vi "SQ Hi--C1.vi"(8 "Command Info In":T2, 10 "Sq. Hi--C1":T1, 11 "Scale":string) -> (0 "Command Info Out":T2)   [LabVIEW 2017]
uses:
  <vilib>/Rock Robotics/WPI/Framework/Command Status Info.ctl
  <vilib>/Rock Robotics/WPI/Framework/Completion Status.ctl
  <vilib>/Rock Robotics/WPI/Framework/Completion Notifier.ctl
  Block Clusters/SQ Hi--C1.ctl
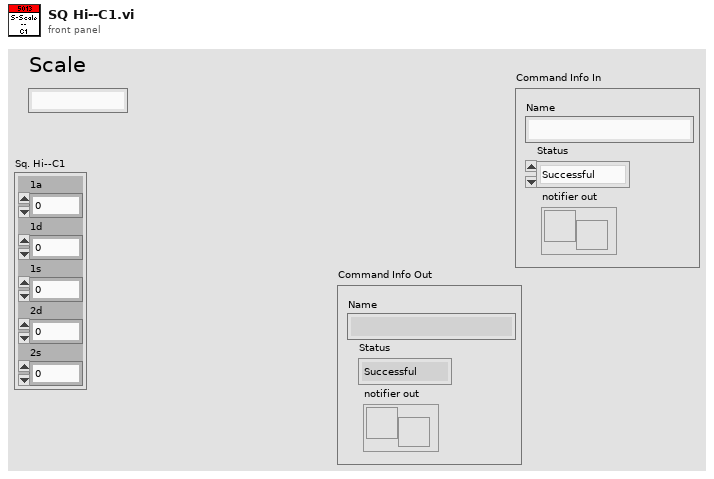
[diagram p1: front panel]
types:
  T1 = typedef "SQ Hi--C1.ctl" = cluster{"1a":dbl, "1d":dbl, "1s":dbl, "2d":dbl, "2s":dbl}
  T2 = typedef "Command Status Info.ctl" = cluster{"Name":string, "Status":T3, "notifier out":T4}
  T3 = typedef "Completion Status.ctl" = enum16{"Successful", "Aborted", "Incomplete"}
  T4 = typedef "Completion Notifier.ctl" = refnum<notifier>
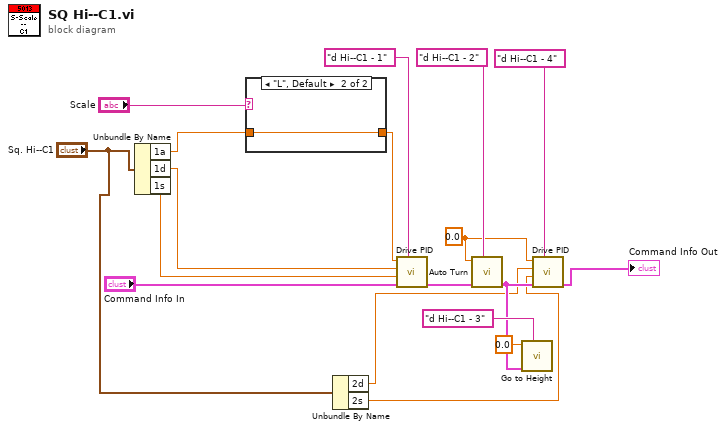
[diagram p0: block diagram]
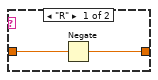
[diagram p2: hidden frame]
diagram:
  w9 = 0.0 ("Target Angle")
  n1 = Unbundle By Name("Sq. Hi--C1") -> ("1a"=w6:dbl, "1d"=w5:dbl, "1s"=w4:dbl)
  n2 = case shown="\"L\", Default" "Scale" {
    tunnel: [w20 w21] -> w18
    tunnel: w6 -> [w19 w21]
    frame "R" {
      n3 = Negate(x=w19) -> (-x=w20:dbl)
    }
    frame "L", Default {
    }
  }
  n4 = Unbundle By Name("Sq. Hi--C1") -> ("2d"=w3:dbl, "2s"=w2:dbl)
  n5 = call "Drive PID.vi"("Description"="d Hi--C1 - 1", "Command Info In"="Command Info In", "Speed"=w4, "Distance"=w5, "Target Angle"=w18) -> ("Command Info Out"=w15:T2)  [unwired: 6 in]
  n6 = call "Auto Turn.vi"("Description"="d Hi--C1 - 2", "Command Info In"=w15, "Target Angle"=w9) -> ("Command Info Out"=w11:T2)  [unwired: 8 in]
  n7 = call "Go to Height.vi"("Description"="d Hi--C1 - 3", "Command Info In"=w11, "Target Height (in)"=0.0) -> ()  [unwired: 8 in, 1 out]
  n8 = call "Drive PID.vi"("Description"="d Hi--C1 - 4", "Command Info In"=w11, "Speed"=w2, "Distance"=w3, "Target Angle"=w9) -> ("Command Info Out"=→"Command Info Out":T2)  [unwired: 6 in]
